vi "Close Plugin Handle.vi"(7 "CIFPluginManager in":refnum<class "CIFPluginManager.lvclass">, 8 "error in (no error)":errorcluster, 11 "Plugin Management Data":T1) -> (0 "error out":errorcluster)   [LabVIEW 2021, in "CIFPluginManager.lvclass"]
uses:
  CIFPluginManager.lvclass
  typedef/Plugin Management Data.ctl
  <vilib>/gRPC/LabVIEW gRPC Library/Shared/grpcId.ctl
  typedef/Loader Type.ctl
  <vilib>/CIF Foundation/CIF Core/CIFCore/Common/Typedef/Version.ctl
  gRPC/CIF_Manager_server/RPC Messages/cif_management_common_PluginStatusData.ctl
  gRPC/CIF_Manager_server/RPC Messages/cif_management_common_PluginStatusData_PluginState.ctl
  gRPC/CIF_Manager_server/RPC Messages/cif_management_common_TimingStatistics.ctl
  gRPC/CIF_Manager_server/RPC Messages/cif_common_TimingStats.ctl
  gRPC/CIF_Manager_server/RPC Messages/cif_management_common_FifoStatistics.ctl
  gRPC/CIF_Manager_server/RPC Messages/cif_management_common_Error.ctl
  gRPC/CIF_Manager_server/RPC Messages/cif_management_common_MonitorDoubles.ctl
  gRPC/CIF_Manager_server/RPC Messages/cif_management_common_MonitorU64.ctl
  gRPC/CIF_Manager_server/RPC Messages/cif_management_common_MonitorI64.ctl
  gRPC/CIF_Manager_server/RPC Messages/cif_management_common_Channels.ctl
  gRPC/CIF_Manager_server/RPC Messages/cif_management_common_Channel.ctl
  gRPC/CIF_Manager_server/RPC Messages/cif_management_common_ChannelDirection.ctl
  gRPC/CIF_Manager_server/RPC Messages/cif_management_common_ChannelPattern.ctl
  CIFPluginManager.lvclass/CIFPluginManager.ctl
  <vilib>/gRPC/LabVIEW gRPC Library/Client API/Close Client.vi
  <vilib>/CIF Foundation/CIF Core/CIFCore/Grpc/CIFCoreWrapper/CIFCoreWrapper.lvlib
  CIFPluginLoader/gRPC/CIF_Plugin_Loader_Client_Wrapper/CIFPluginLoaderClientWrapper.lvlib
  <vilib>/CIF Foundation/CIF Core/CIFCore/Common/CIFCoreCommon.lvlib
  <vilib>/gRPC/LabVIEW gRPC Library/grpc-lvsupport-release.lvlib
  gRPC/CIF_Manager_server/CIF_Manager_server.lvlib
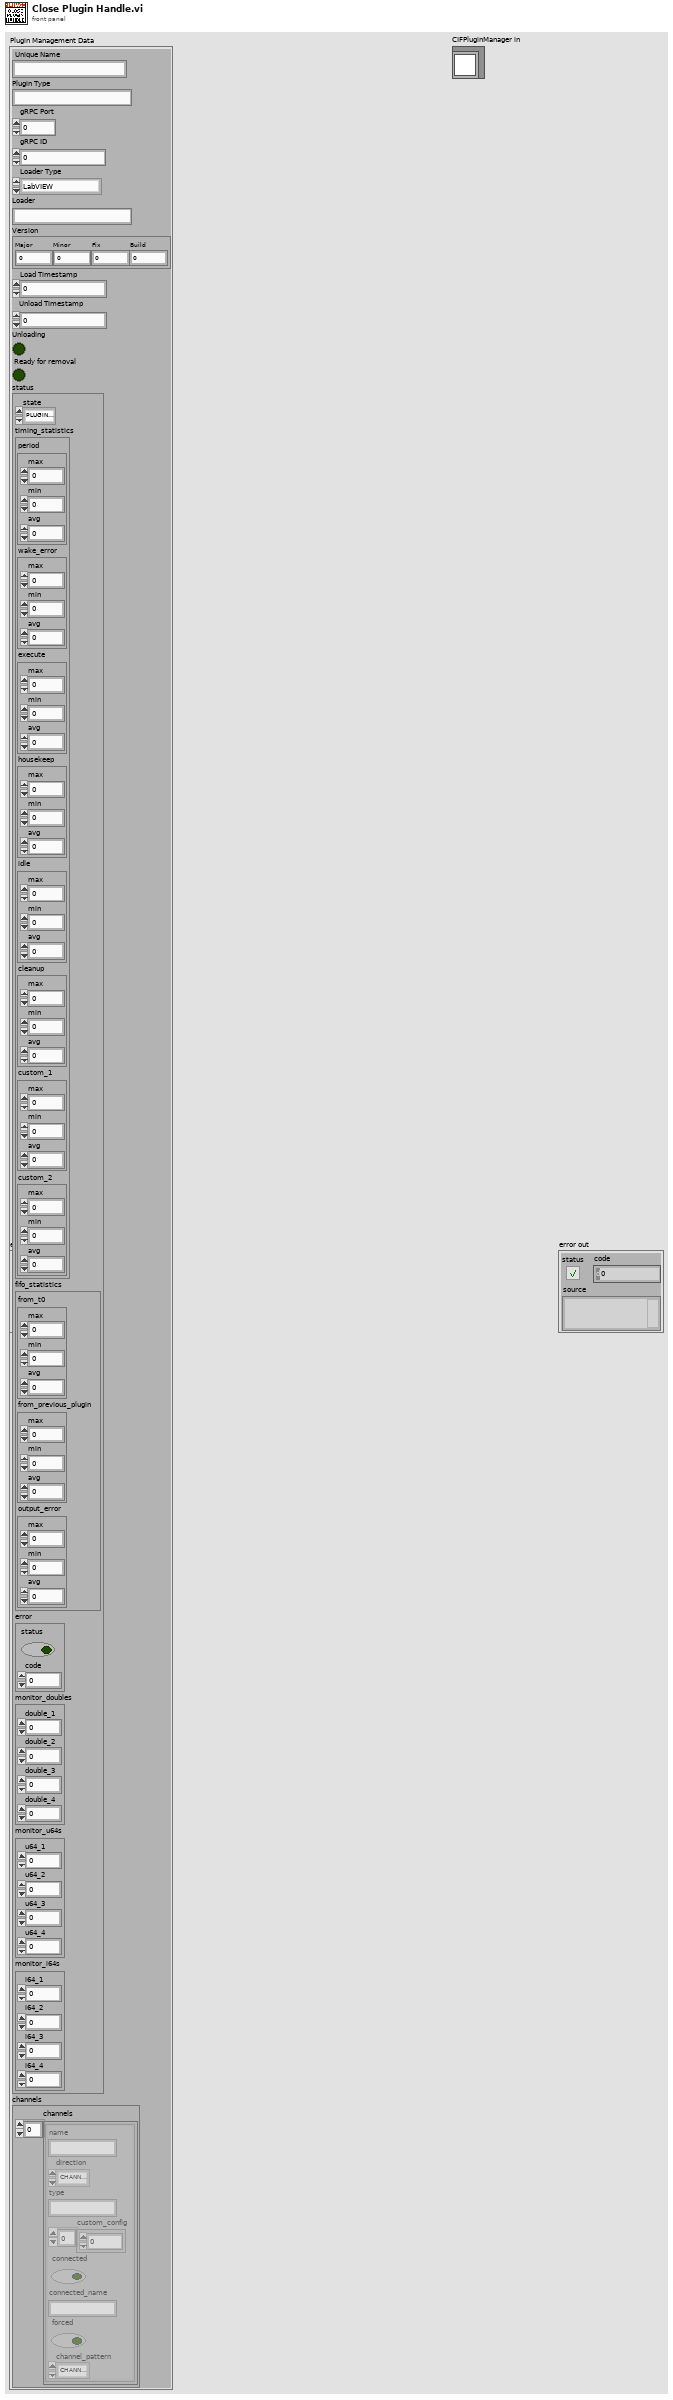
[diagram p1: front panel]
types:
  T1 = typedef "CIFPluginManager.lvclass/Plugin Management Data.ctl" = cluster{"Unique Name":string, "Plugin Type":string, "gRPC Port":i32, "gRPC ID":T2, "Loader Type":T3, "Loader":string, "Version":T4, "Load Timestamp":i64, "Unload Timestamp":i64, "Unloading":bool, "Ready for removal":bool, "status":T5, "channels":T14}
  T2 = typedef "grpc-lvsupport-release.lvlib/grpcId.ctl" = u64
  T3 = typedef "CIFPluginManager.lvclass/Loader Type.ctl" = enum16{"LabVIEW"}
  T4 = typedef "CIFCoreCommon.lvlib/Version.ctl" = cluster{"Major":i32, "Minor":i32, "Fix":i32, "Build":i32}
  T5 = typedef "CIF_Manager_server.lvlib/cif_management_common_PluginStatusData.ctl" = cluster{"state":T6, "timing_statistics":T7, "fifo_statistics":T9, "error":T10, "monitor_doubles":T11, "monitor_u64s":T12, "monitor_i64s":T13}
  T6 = typedef "CIF_Manager_server.lvlib/cif_management_common_PluginStatusData_PluginState.ctl" = enum32{"PLUGINSTATE_UNKNOWN", "PLUGINSTATE_CREATING", "PLUGINSTATE_LISTENING", "PLUGINSTATE_RUNNING", "PLUGINSTATE_CLEANINGUP", "PLUGINSTATE_DESTROYING"}
  T7 = typedef "CIF_Manager_server.lvlib/cif_management_common_TimingStatistics.ctl" = cluster{"period":T8, "wake_error":T8, "execute":T8, "housekeep":T8, "idle":T8, "cleanup":T8, "custom_1":T8, "custom_2":T8}
  T8 = typedef "CIF_Manager_server.lvlib/cif_common_TimingStats.ctl" = cluster{"max":i64, "min":i64, "avg":dbl}
  T9 = typedef "CIF_Manager_server.lvlib/cif_management_common_FifoStatistics.ctl" = cluster{"from_t0":T8, "from_previous_plugin":T8, "output_error":T8}
  T10 = typedef "CIF_Manager_server.lvlib/cif_management_common_Error.ctl" = cluster{"status":bool, "code":i32}
  T11 = typedef "CIF_Manager_server.lvlib/cif_management_common_MonitorDoubles.ctl" = cluster{"double_1":dbl, "double_2":dbl, "double_3":dbl, "double_4":dbl}
  T12 = typedef "CIF_Manager_server.lvlib/cif_management_common_MonitorU64.ctl" = cluster{"u64_1":u64, "u64_2":u64, "u64_3":u64, "u64_4":u64}
  T13 = typedef "CIF_Manager_server.lvlib/cif_management_common_MonitorI64.ctl" = cluster{"i64_1":i64, "i64_2":i64, "i64_3":i64, "i64_4":i64}
  T14 = typedef "CIF_Manager_server.lvlib/cif_management_common_Channels.ctl" = cluster{"channels":T15[]}
  T15 = typedef "CIF_Manager_server.lvlib/cif_management_common_Channel.ctl" = cluster{"name":string, "direction":T16, "type":string, "custom_config":u8[], "connected":bool, "connected_name":string, "forced":bool, "channel_pattern":T17}
  T16 = typedef "CIF_Manager_server.lvlib/cif_management_common_ChannelDirection.ctl" = enum32{"CHANNELDIRECTION_UNKNOWN", "CHANNELDIRECTION_PUBLISHER", "CHANNELDIRECTION_SUBSCRIBER"}
  T17 = typedef "CIF_Manager_server.lvlib/cif_management_common_ChannelPattern.ctl" = enum32{"CHANNELPATTERN_UNKNOWN", "CHANNELPATTERN_TAG", "CHANNELPATTERN_FIFO", "CHANNELPATTERN_MULTIFIFO", "CHANNELPATTERN_BACKPRESSUREFIFO"}
  T18 = typedef "CIFPluginManager.lvclass/Loader Map.ctl" = map{string, T19}
  T19 = typedef "CIFPluginManager.lvclass/Loaders.ctl" = cluster{"Loader Type":T3, "grpc_port":i32, "pid":u32, "gRPC ID":T2, "Load Timestamp":i64, "Unloading":bool, "Ready for removal":bool, "Unload Timestamp":i64}
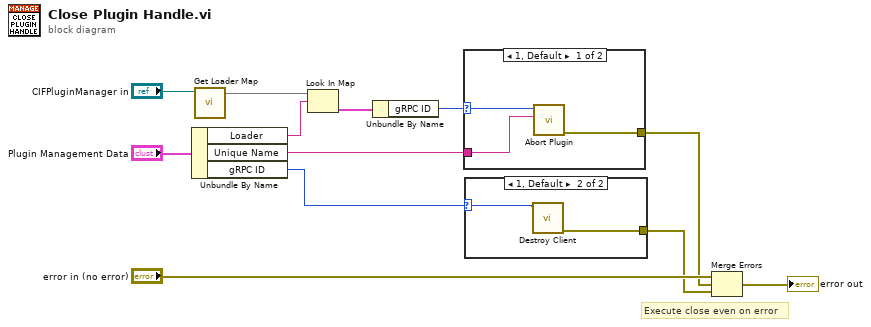
[diagram p0: block diagram]
diagram:
  # "Execute close even on error"
  n1 = Unbundle By Name("Plugin Management Data") -> ("Loader"=w4:string, "Unique Name"=w2:string, "gRPC ID"=w8:T2)
  n2 = call "Get Loader Map.vi"("CIFPluginManager in"="CIFPluginManager in") -> ("Loader Map"=w5:T18)  [unwired: 9 in, 1 out]
  n3 = Look In Map(map=w5, key=w4) -> (value=w3:T19)  [unwired: 1 in, 1 out]
  n4 = Unbundle By Name(w3) -> ("gRPC ID"=w1:T2)
  n5 = case shown="1, Default" w1 {
    selector: w1 -> [w13 _]
    tunnel: [w14 _] -> w11
    tunnel: w2 -> [w15 _]
    frame 1, Default {
      n6 = call "Abort Plugin.vi"("plugin_name"=w15, "gRPC ID in"=w13) -> ("error out"=w14:errorcluster)  [unwired: 8 in, 1 out]
    }
    frame 0 {
    }
  }
  n7 = case shown="1, Default" w8 {
    selector: w8 -> [_ w17]
    tunnel: [_ w16] -> w9
    frame 0 {
    }
    frame 1, Default {
      n8 = call <vilib>:"Destroy Client.vi"("gRPC ID"=w17) -> ("error out"=w16:errorcluster)  [unwired: 10 in]
    }
  }
  n9 = Merge Errors("error in (no error)", w11, w9) -> (→"error out":errorcluster)
